vi "Config Aout Bias.vi"(8 "error in":errorcluster, 9 "Loss (1.0 V)":dbl=1.0 min=-10.5 max=10.5 format="%#_6f", 10 "Capacitance (1.0 V)":dbl=1.0 min=-10.5 max=10.5 format="%#_6f", 11 "VISA resource name":refnum<visa-resource-name>) -> (0 "error out":errorcluster, 3 "VISA resource name out":refnum<visa-resource-name>)   [LabVIEW 2019, in "Andeen-Hagerling 2700(400 firmware).lvlib"]
doc: "Sets the output level produced by the capacitance and/or loss bias voltage sources."
uses:
  Andeen-Hagerling 2700(400 firmware).lvlib
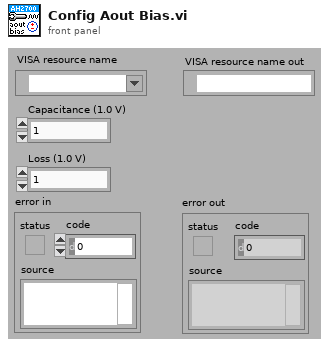
[diagram p1: front panel]
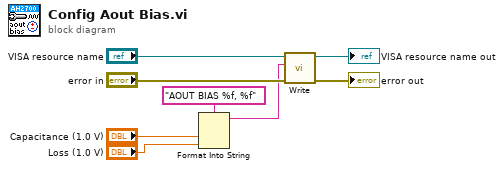
[diagram p0: block diagram]
diagram:
  n1 = Format Into String(format string="AOUT BIAS %f, %f", "Capacitance (1.0 V)", "Loss (1.0 V)") -> (resulting string=w1:string)  [unwired: 2 in, 1 out]
  n2 = call "Write.vi"("error in"="error in", "command"=w1, "VISA resource name"="VISA resource name") -> ("error out"=→"error out":errorcluster, "VISA resource name out"=→"VISA resource name out":refnum<visa-resource-name>)  [unwired: 7 in]
